vi "Retrieve_GetTargetImageInfo.vi"(8 "error in (no error)":errorcluster, 11 "DevInfo":T3={"Hostname"="", "IPAddress"="", "MAC"="", "SerialNum"="", "Model"="", "Status"="", "FW"="", "OSDesc"="", "ImgTitle"="", "ImgDesc"="", "ImgVer"="", "ImgID"="", "IP Address Request Mode"=1, "SubnetMask"="", "Gateway"="", "DNSServer"=""} {"IP Address Request Mode" items=["Static"=1, "DHCP/Link-Local"=2, "Link-Local Only"=4, "DHCP Only"=8]}) -> (0 "error out":errorcluster, 2 "Supports SysCfg Metadata":bool, 3 "AppImage Properties":T1)   [LabVIEW 2021]
uses:
  TypeDefs/DevInfo.ctl
  TypeDefs/AppImageProperties.ctl
  TypeDefs/FPGA_Properties_Element.ctl
  TypeDefs/TargetAccess.ctl
  <vilib>/nisyscfg/Close (System).vi
  <resource>/objmgr/nisysapi.rc
  <vilib>/nisyscfg/nisyscfg.lvlib
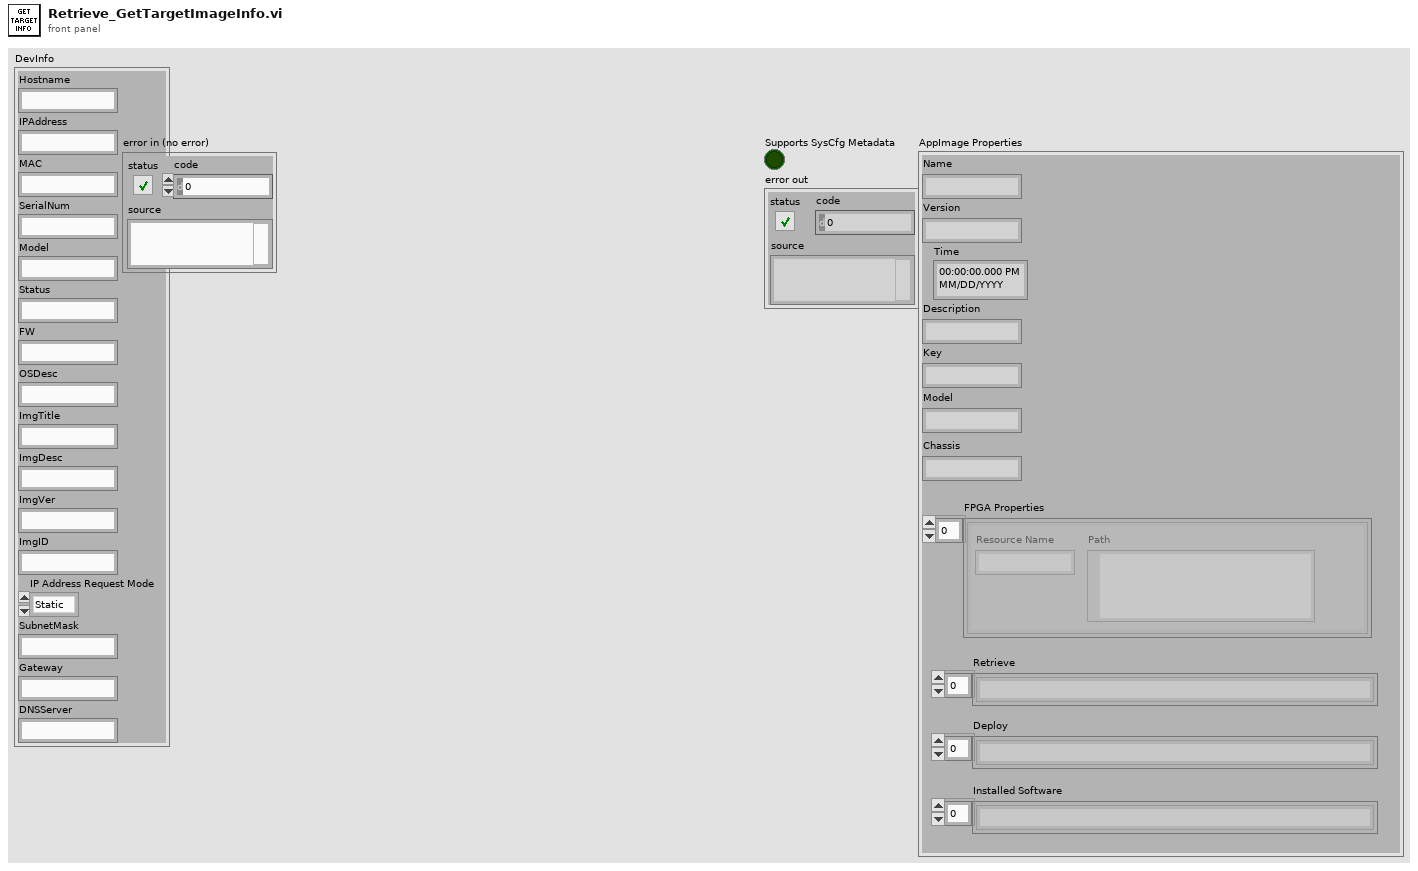
[diagram p1: front panel]
types:
  T1 = typedef "AppImageProperties.ctl" = cluster{"Name":string, "Version":string, "Time":timestamp, "Description":string, "Key":string, "Chassis":string, "FPGA Properties":T2[], "Model":string, "Retrieve":string[], "Deploy":string[], "Installed Software":string[]}
  T2 = typedef "FPGA_Properties_Element.ctl" = cluster{"Resource Name":string, "Path":path}
  T3 = typedef "DevInfo.ctl" = cluster{"Hostname":string, "IPAddress":string, "MAC":string, "SerialNum":string, "Model":string, "Status":string, "FW":string, "OSDesc":string, "ImgTitle":string, "ImgDesc":string, "ImgVer":string, "ImgID":string, "IP Address Request Mode":i32, "SubnetMask":string, "Gateway":string, "DNSServer":string}
  T4 = typedef "TargetAccess.ctl" = enum16{"Read-Only", "Admin"}
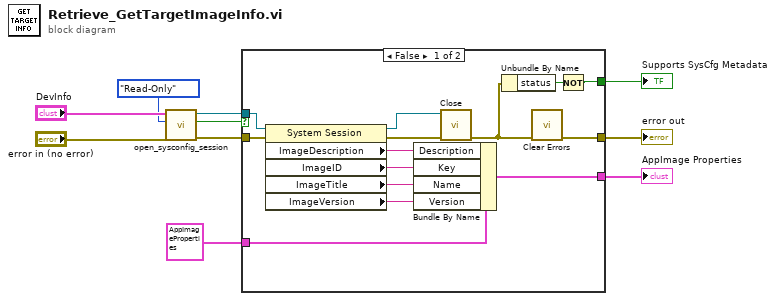
[diagram p0: block diagram]
diagram:
  n1 = call "open_sysconfig_session.vi"("error in (no error)"="error in (no error)", "Target Access"=TargetAccess."Read-Only", "DevInfo"="DevInfo") -> ("error out"=w5:errorcluster, "Cancelled"=w8:bool, "Session Out"=w6:refnum<k21>)  [unwired: 6 in]
  n2 = case shown="False" w8 {
    tunnel: T1 {"Name"="", "Version"="", "Time"=timestamp(0 s since 1904-01-01), "Description"="", "Key"="", "Chassis"="", "FPGA Properties"=[], "Model"="", "Retrieve"=[], "Deploy"=[], "Installed Software"=[]} ("AppImage Properties") -> [w15 w25]
    tunnel: w6 -> [w11 _]
    tunnel: w5 -> [w16 w26]
    tunnel: [w14 w25] -> w2
    tunnel: [w13 _] -> w4
    tunnel: [w12 w26] -> w3
    frame False {
      n3 = property class="System Session"(reference=w11, error in=w16) -> (reference out=w21:refnum<k21>, error out=w20:errorcluster, "ImageDescription"=w17:string, "ImageID"=w22:string, "ImageTitle"=w18:string, "ImageVersion"=w19:string)
      n4 = Bundle By Name(cluster=w15, "Description"=w17, "Key"=w22, "Name"=w18, "Version"=w19) -> (w14:T1)
      n5 = call-poly <vilib>:"Close.vi"("error in (no error)"=w20, "Session in"=w21) -> ("error out"=w23:errorcluster)  [unwired: 9 in]
      n6 = Unbundle By Name(w23) -> ("status"=w24:bool)
      n7 = call <vilib>:"Clear Errors.vi"("error in (no error)"=w23) -> ("error out"=w12:errorcluster)  [unwired: 5 in, 1 out]
      n8 = Not(x=w24) -> (.not. x?=w13:bool)
    }
    frame True {
    }
  }
  "Supports SysCfg Metadata" <- w4
  "error out" <- w3
  "AppImage Properties" <- w2
